vi "Taiko_ProcCmd.vi"(8 "Cmd in":T1=enum."Init", 11 "Data in":T2 {"TaggedValueList"."Tag" format="%x" items=["NONE"=0, "Locked"=16, "SoftLock"=17, "KeyLock"=18, "Class_IV_Lock"=20, "Interlock"=24, "LaserMode"=32, "LDH_PulsePowerTable"=33, "TriggerMode"=48, "TriggerLevelRaw"=64, "TriggerLevelRawLoLimit"=65, "TriggerLevelRawHiLimit"=66, "TriggerLevel"=72, "TriggerLevelLoLimit"=73, "TriggerLevelHiLimit"=74, "FastGate"=80, "FastGateImp"=96, "SlowGate"=112, "TargetTempRaw"=144, "TargetTempRawLoLimit"=145, "TargetTempRawHiLimit"=146, "CurrentTempRaw"=148, "CaseTempRaw"=149, "TargetTemp"=152, "TargetTempLoLimit"=153, "TargetTempHiLimit"=154, "CurrentTemp"=156, "CaseTemp"=157, "TempScale"=159, "Frequency"=168, "FrequencyLoLimit"=169, "FrequencyHiLimit"=170, "PulsePowerRaw"=176, "PulsePowerRawLoLimit"=177, "PulsePowerRawHiLimit"=178, "PulsePowerPermille"=180, "PulseShape"=181, "PulsePower"=184, "PulsePowerLoLimit"=185, "PulsePowerHiLimit"=186, "PulsePowerNanowatt"=188, "PulsePowerVoltage"=190, "PulseEnergy"=191, "CwPowerRaw"=192, "CwPowerRawLoLimit"=193, "CwPowerRawHiLimit"=194, "CwPowerPermille"=196, "CwPower"=200, "CwPowerLoLimit"=201, "CwPowerHiLimit"=202, "CwPowerMicroWatt"=204, "BurstLen"=208, "BurstPeriod"=224, "LDH_Fan"=240, "UI_Exclusive"=256]}) -> (0 "Cmd out":T1=enum."Init", 2 "Cmd prev":T1=enum."Init", 3 "Data out":T2 {"TaggedValueList"."Tag" format="%x" items=["NONE"=0, "Locked"=16, "SoftLock"=17, "KeyLock"=18, "Class_IV_Lock"=20, "Interlock"=24, "LaserMode"=32, "LDH_PulsePowerTable"=33, "TriggerMode"=48, "TriggerLevelRaw"=64, "TriggerLevelRawLoLimit"=65, "TriggerLevelRawHiLimit"=66, "TriggerLevel"=72, "TriggerLevelLoLimit"=73, "TriggerLevelHiLimit"=74, "FastGate"=80, "FastGateImp"=96, "SlowGate"=112, "TargetTempRaw"=144, "TargetTempRawLoLimit"=145, "TargetTempRawHiLimit"=146, "CurrentTempRaw"=148, "CaseTempRaw"=149, "TargetTemp"=152, "TargetTempLoLimit"=153, "TargetTempHiLimit"=154, "CurrentTemp"=156, "CaseTemp"=157, "TempScale"=159, "Frequency"=168, "FrequencyLoLimit"=169, "FrequencyHiLimit"=170, "PulsePowerRaw"=176, "PulsePowerRawLoLimit"=177, "PulsePowerRawHiLimit"=178, "PulsePowerPermille"=180, "PulseShape"=181, "PulsePower"=184, "PulsePowerLoLimit"=185, "PulsePowerHiLimit"=186, "PulsePowerNanowatt"=188, "PulsePowerVoltage"=190, "PulseEnergy"=191, "CwPowerRaw"=192, "CwPowerRawLoLimit"=193, "CwPowerRawHiLimit"=194, "CwPowerPermille"=196, "CwPower"=200, "CwPowerLoLimit"=201, "CwPowerHiLimit"=202, "CwPowerMicroWatt"=204, "BurstLen"=208, "BurstPeriod"=224, "LDH_Fan"=240, "UI_Exclusive"=256]})   [LabVIEW 2010]
uses:
  Types/Taiko_Cmds.ctl
  Types/Taiko_Data.ctl
  _lib/PDLM/pdlm_lib_x86_x64_UIThread.llb/PDLM_Tag.ctl
  _lib/PDLM/pdlm_lib_x86_x64_UIThread.llb/PDLM_TaggedValue.ctl
  _lib/PDLM/pdlm_lib_x86_x64_UIThread.llb/PDLM_TaggedValueList.ctl
  Types/ControlAttributes.ctl
  Types/ScaleDisplayParams.ctl
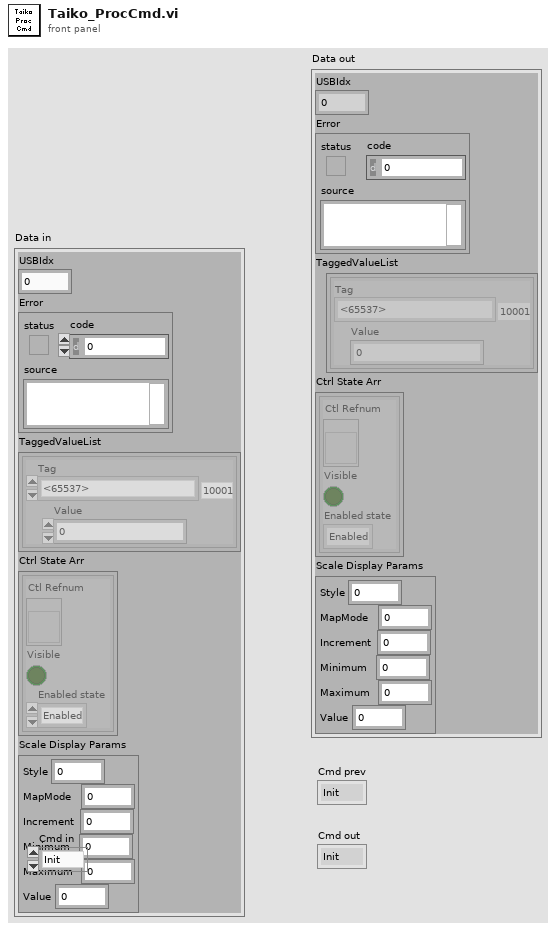
[diagram p1: front panel]
types:
  T1 = typedef "Taiko_Cmds.ctl" = enum16{"Idle", "Init", "Exit", "Update", "Error"}
  T2 = typedef "Taiko_Data.ctl" = cluster{"USBIdx":i32, "Error":errorcluster, "TaggedValueList":T3, "Ctrl State Arr":T6[], "Scale Display Params":T7}
  T3 = typedef "PDLM_TaggedValueList.ctl" = T4[]
  T4 = typedef "PDLM_TaggedValue.ctl" = cluster{"Tag":T5, "Value":u32}
  T5 = typedef "PDLM_Tag.ctl" = u32
  T6 = typedef "ControlAttributes.ctl" = cluster{"Ctl Refnum":refnum<vi>, "Visible":bool, "Enabled state":enum8{"Enabled", "Disabled", "Disabled and Grayed Out"}}
  T7 = typedef "ScaleDisplayParams.ctl" = cluster{"Style":u8, "MapMode":u8, "Increment":dbl, "Minimum":dbl, "Maximum":dbl, "Value":dbl}
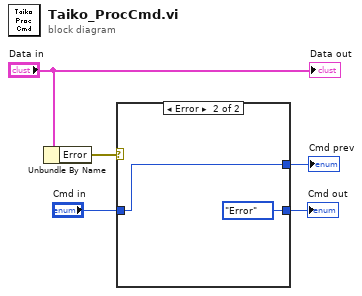
[diagram p0: block diagram]
diagram:
  n1 = Unbundle By Name("Data in") -> ("Error"=w5:errorcluster)
  n2 = case shown="Error" w5 {
    tunnel: [w6 Taiko_Cmds."Error" ("Cmd in")] -> w3
    tunnel: "Cmd in" -> [w6 w7]
    tunnel: [_ w7] -> w1
    frame No Error {
    }
    frame Error {
    }
  }
  "Cmd out" <- w3
  "Cmd prev" <- w1
  "Data out" <- "Data in"
